vi "GetMFCSetPoints.vi"() -> ()   [LabVIEW 2011]
panel:
  out "SetPoints":dbl[](array[numeric])
  in  "Indices":i32[](array[numeric])
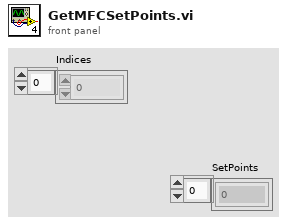
[diagram p1: front panel]
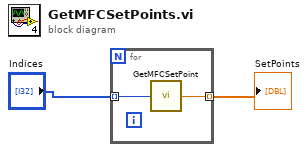
[diagram p0: block diagram]
diagram:
  n1 = for {
    tunnel: "Indices" -> [w4] mode=indexing
    tunnel: [w3] -> w1 mode=indexing
    n2 = call "GetMFCSetPoint.vi"("MFC ID Number"=w4) -> ("SetPoint"=w3:dbl)
  }
  "SetPoints" <- w1
